vi "Overlay Image with Sector ROI.vi"(7 "FPGA Display Image In":T1=refnum, 8 "error in":errorcluster, 11 "FPGA Image":T1=refnum) -> (0 "error out":errorcluster, 3 "FPGA Display Image Out":T1)   [LabVIEW 2013]
uses:
  <vilib>/vision/Image Controls.llb/IMAQ Image.ctl
  Image Processing/Mask ROI FG Enum.ctl
  Globals/Average Sector Data.vi
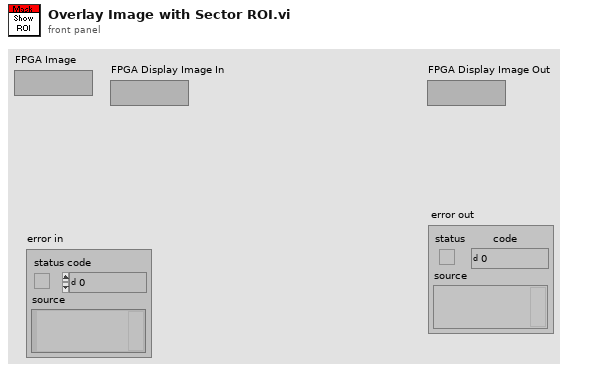
[diagram p1: front panel]
types:
  T1 = typedef "IMAQ Image.ctl" = refnum<image>
  T2 = typedef "Mask ROI FG Enum.ctl" = enum16{"Read", "Write"}
  T3 = typedef "Mask ROI Cluster.ctl" = cluster{"left annulus":T4, "right annulus":T4, "Threshold Range":cluster{"Lower value":dbl, "Upper value":dbl}, "[Avg BG]":u8[], "Number of Sectors":u8, "Left ROI":T5, "Right ROI":T5, "Left Start Angle Duty Cycle":fxp<+,8,0>, "Left End Angle Duty Cycle":fxp<+,8,0>, "Right End Angle Duty Cycle":fxp<+,8,0>, "Right Start Angle Duty Cycle":fxp<+,8,0>, "[Sector ROIs]":T5[]}
  T4 = typedef "IMAQ Circle" = cluster{"Center X":i32, "Center Y":i32, "Inner Radius":i32, "Outer Radius":i32, "Start Angle":dbl, "End Angle":dbl}
  T5 = typedef "ROI Descriptor" = cluster{"Global Rectangle":i32[], "Contours":cluster{"ID":enum32{"External", "Internal"}, "Type":u32, "Coordinates":i32[]}[]}
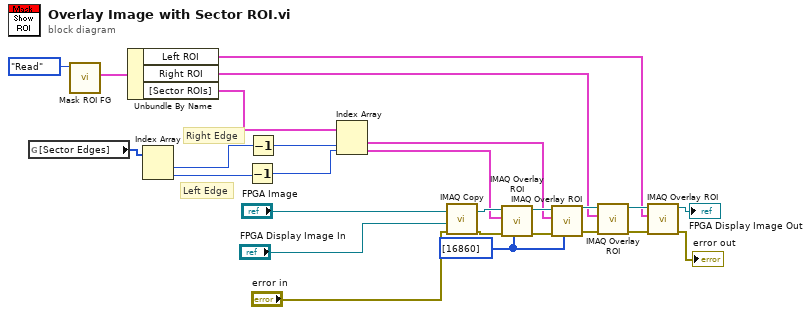
[diagram p0: block diagram]
diagram:
  w1 = u32[] [16860] ("Colors (Green)")
  # "Left Edge"
  # "Right Edge"
  n1 = global read "Average Sector Data.vi" "[Sector Edges]"() -> (w4:u8[])
  n2 = call "Mask ROI FG.vi"("Operation"=Mask_ROI_FG_Enum."Read") -> ("Mask ROI Out"=w9:T3)  [unwired: 9 in, 1 out]
  n3 = Unbundle By Name(w9) -> ("Left ROI"=w8:T5, "Right ROI"=w7:T5, "[Sector ROIs]"=w6:T5[])
  n4 = Index Array(array=w4) -> (element #1=w2:u8, element #2=w3:u8)  [unwired: 2 in]
  n5 = Decrement(x=w3) -> (x-1=w18:u8)
  n6 = Decrement(x=w2) -> (x-1=w19:u8)
  n7 = Index Array(array=w6, index #1=w19, index #2=w18) -> (element #1=w10:T5, element #2=w11:T5)
  n8 = call "IMAQ Copy"("error in (no error)"="error in", "Image Dst"="FPGA Display Image In", "Image Src"="FPGA Image") -> ("error out"=w22:errorcluster, "Image Dst Out"=w26:T1)  [unwired: 3 in]
  n9 = call "IMAQ Overlay ROI"("Colors (Green)"=w1, "error in (no error)"=w22, "ROI Descriptor"=w11, "Image"=w26) -> ("error out"=w25:errorcluster, "Image Out"=w24:T1)  [unwired: 6 in]
  n10 = call "IMAQ Overlay ROI"("Colors (Green)"=w1, "error in (no error)"=w25, "ROI Descriptor"=w10, "Image"=w24) -> ("error out"=w12:errorcluster, "Image Out"=w16:T1)  [unwired: 6 in]
  n11 = call "IMAQ Overlay ROI"("error in (no error)"=w12, "ROI Descriptor"=w7, "Image"=w16) -> ("error out"=w17:errorcluster, "Image Out"=w15:T1)  [unwired: 7 in]
  n12 = call "IMAQ Overlay ROI"("error in (no error)"=w17, "ROI Descriptor"=w8, "Image"=w15) -> ("error out"=→"error out":errorcluster, "Image Out"=→"FPGA Display Image Out":T1)  [unwired: 7 in]
